vi "Digital_Read.vi"(8 "error in (no error)":errorcluster, 10 "Pin":u8=4 min=4 max=40, 11 "VISA resource name":refnum<visa-resource-name>) -> (0 "error out":errorcluster, 2 "Valor":bool, 3 "VISA resource name out":refnum<visa-resource-name>)   [LabVIEW 2025]
doc: "Este VI permite enviar una instruccion de lectura digital al pin elegido \nDebe recibir los datos de VISA resource name, Error IN y el pin a leer\nDara como salida VISA resource name, estado logico de lectura y error OUT"
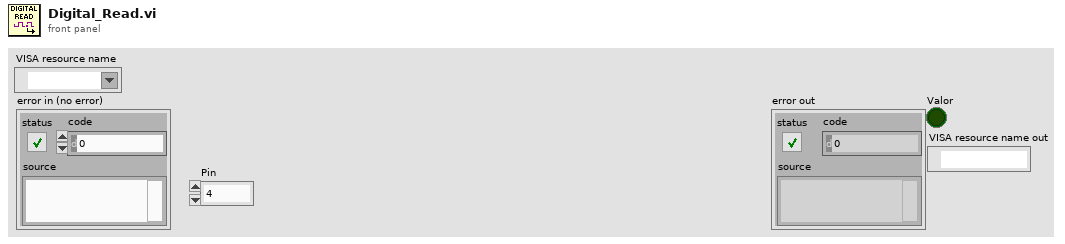
[diagram p1: front panel]
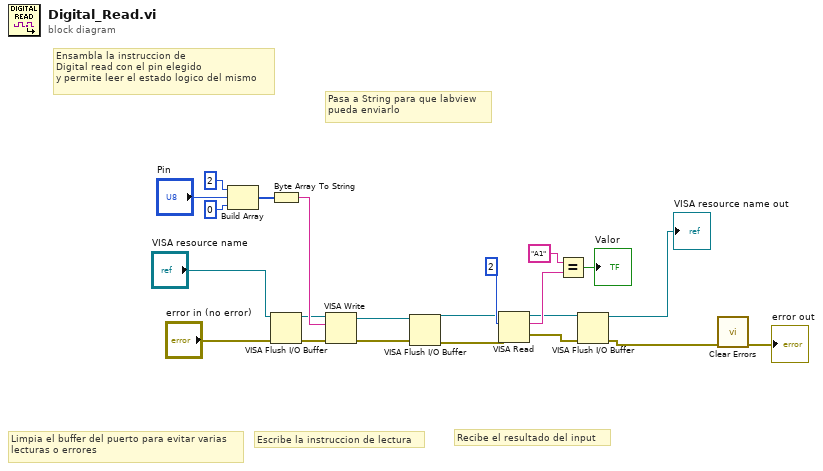
[diagram p0: block diagram]
diagram:
  # "Recibe el resultado del input"
  # "Escribe la instruccion de lectura"
  # "Limpia el buffer del puerto para evitar varias\nlecturas o errores"
  # "Pasa a String para que labview \npueda enviarlo"
  # "Ensambla la instruccion de \nDigital read con el pin elegido\ny permite leer el estado logico del mismo"
  n1 = Build Array(u8 2, "Pin", u8 0) -> (w20:u8[])
  n2 = Byte Array To String(unsigned byte array=w20) -> (string=w22:string)
  n3 = VISA Flush I/O Buffer(VISA resource name="VISA resource name", error in (no error)="error in (no error)") -> (VISA resource name out=w14:refnum<visa-resource-name>, error out=w13:errorcluster)  [unwired: 1 in]
  n4 = VISA Write(VISA resource name=w14, write buffer=w22, error in (no error)=w13) -> (VISA resource name out=w2:refnum<visa-resource-name>, error out=w1:errorcluster)  [unwired: 1 out]
  n5 = VISA Flush I/O Buffer(VISA resource name=w2, error in (no error)=w1) -> (VISA resource name out=w3:refnum<visa-resource-name>, error out=w4:errorcluster)  [unwired: 1 in]
  n6 = VISA Read(VISA resource name=w3, byte count=u32 2, error in (no error)=w4) -> (VISA resource name out=w7:refnum<visa-resource-name>, read buffer=w17:string, error out=w8:errorcluster)  [unwired: 1 out]
  n7 = Equal?(x="A1", y=w17) -> (x = y?=→"Valor":bool)
  n8 = VISA Flush I/O Buffer(VISA resource name=w7, error in (no error)=w8) -> (VISA resource name out=→"VISA resource name out":refnum<visa-resource-name>, error out=w9:errorcluster)  [unwired: 1 in]
  n9 = call <vilib>:"Clear Errors.vi"("error in (no error)"=w9) -> ("error out"=→"error out":errorcluster)  [unwired: 5 in, 1 out]
